vi "Config Marker Polarity.vi"(0 "VISA Resource Name":refnum<visa-resource-name>, 1 "Standard (0: IS-95A)":T1(ring), 2 "Marker (0: Marker 1)":u16(ring) items=["Marker 1", "Marker 2", "Marker 3", "Marker 4"], 3 "Polarity (0: Negative)":enum16{"Negative", "Positive"}(ring), 5 "error in (no error)":errorcluster {"code" format="%.0x"}) -> (14 "VISA Resource Name Out":refnum<visa-resource-name>, 19 "error out":errorcluster {"code" format="%.0x"})   [LabVIEW 2014, in "Agilent ESG Series.lvlib"]
doc: "This VI Sets the polarity for selected marker.\n\nNotes:\n(1) This VI is valid only on instrument E4438C."
uses:
  Agilent ESG Series.lvlib
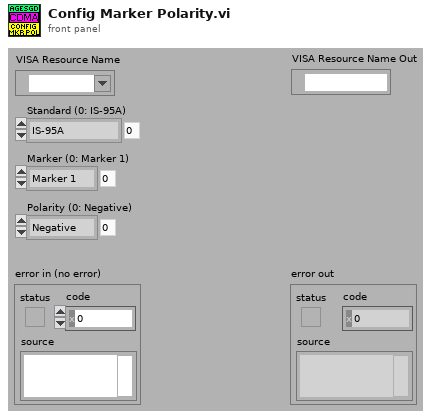
[diagram p1: front panel]
types:
  T1 = enum16{"IS-95A", "CDMA2000", "WCDMA", "Dual Arbitrary"}
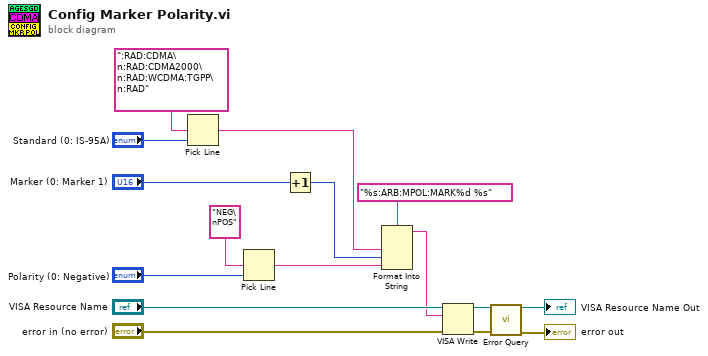
[diagram p0: block diagram]
diagram:
  n1 = Pick Line(multi-line string=":RAD:CDMA\n:RAD:CDMA2000\n:RAD:WCDMA:TGPP\n:RAD", line index="Standard (0: IS-95A)") -> (output string=w4:string)  [unwired: 1 in]
  n2 = Pick Line(multi-line string="NEG\nPOS", line index="Polarity (0: Negative)") -> (output string=w5:string)  [unwired: 1 in]
  n3 = Increment(x="Marker (0: Marker 1)") -> (x+1=w1:u16)
  n4 = Format Into String(format string="%s:ARB:MPOL:MARK%d %s", w4, w1, w5) -> (resulting string=w2:string)  [unwired: 2 in, 1 out]
  n5 = VISA Write(VISA resource name="VISA Resource Name", write buffer=w2, error in (no error)="error in (no error)") -> (VISA resource name out=w12:refnum<visa-resource-name>, error out=w11:errorcluster)  [unwired: 1 out]
  n6 = call "Error Query.vi"("VISA Resource Name"=w12, "error in (no error)"=w11) -> ("VISA Resource Name Out"=→"VISA Resource Name Out":refnum<visa-resource-name>, "error out"=→"error out":errorcluster)  [unwired: 10 in, 2 out]
